vi "Batch Load Data.vi"(8 "Y Array Input":dbl[][](array[numeric])=array1024x10[10240 elements] format="%.2f") -> (2 "Data Array output":dbl[][](array[numeric])=[[156320.0], [157260.0], [158740.0], [160150.0], [162530.0], [164140.0], [166060.0], [167590.0], [169200.0], [171260.0], [172690.0], [174810.0], [176260.0], [178620.0], [180480.0], [181740.0], [183460.0], [185700.0], [187270.0], [189260.0], [191040.0], [192940.0], [193980.0], [196750.0], [198840.0], [200170.0], [202190.0], [203860.0], [205040.0], [206430.0], [209340.0], [210440.0], [213240.0], [214740.0], [216720.0], [218710.0], [220610.0], [222540.0], [224090.0], [226040.0], [227760.0], [228770.0], [231810.0], [233660.0], [235500.0], [237390.0], [239590.0], [241700.0], [243190.0], [245260.0], [245670.0], [248540.0], [250180.0], [252160.0], [254040.0], [255810.0], [257360.0], [258980.0], [260540.0], [261970.0], [262240.0], [265810.0], [266800.0], [268760.0], [270660.0], [271180.0], [273130.0], [274420.0], [276410.0], [276090.0], [278520.0], [280230.0], [281030.0], [281870.0], [283440.0], [285750.0], [286320.0], [287530.0], [288750.0], [288670.0], [290950.0], [292320.0], [293710.0], [294870.0], [295370.0], [296240.0], [297700.0], [298710.0], [298800.0], [301150.0], [302130.0], [303180.0], [303690.0], [304680.0], [305540.0], [306660.0], [307720.0], [308220.0], [307800.0], [310510.0], [310980.0], [311540.0], [312460.0], [312990.0], [313790.0], [314260.0], [315080.0], [314160.0], [316990.0], [317280.0], [317390.0], [317810.0], [318990.0], [319270.0], [319920.0], [320880.0], [320580.0], [321670.0], [323440.0], [324260.0], [324090.0], [325340.0], [326440.0], [327880.0], [328190.0], [329450.0], [328800.0], [331840.0], [332880.0], [333390.0], [334690.0], [335400.0], [336540.0], [337530.0], [338800.0], [338680.0], [340000.0], [341080.0], [341600.0], [342840.0], [343390.0], [344390.0], [345420.0], [346090.0], [346340.0], [346460.0], [349550.0], [349420.0], [350670.0], [351070.0], [351930.0], [353120.0], [353520.0], [354520.0], [354640.0], [355380.0], [356380.0], [357290.0], [358190.0], [358930.0], [359670.0], [359540.0], [360830.0], [361900.0], [360600.0], [362480.0], [363660.0], [364070.0], [364740.0], [364990.0], [366060.0], [366930.0], [367780.0], [367940.0], [368640.0], [369950.0], [370430.0], [371320.0], [371730.0], [372740.0], [373400.0], [373890.0], [374850.0], [374640.0], [376240.0], [378000.0], [377860.0], [379380.0], [380050.0], [380630.0], [381640.0], [382180.0], [382230.0], [383250.0], [385270.0], [385380.0], [387220.0], [387590.0], [387980.0], [389810.0], [390380.0], [391030.0], [390020.0], [392370.0], [393610.0], [394220.0], [394720.0], [395770.0], [397090.0], [397800.0], [398480.0], [398130.0], [399860.0], [400870.0], [401860.0], [402070.0], [403020.0], [404320.0], [405070.0], [406210.0], [407160.0], [406140.0], [408920.0], [410760.0], [410970.0], [412260.0], [413420.0], [414890.0], [415800.0], [416960.0], [417480.0], [417970.0], [420910.0], [421760.0], [422450.0], [425020.0], [425520.0], [427330.0], [429060.0], [430200.0], [429790.0], [433380.0], [434550.0], [435800.0], [437460.0], [439590.0], [441200.0], [442140.0], [444010.0], [444080.0], [447490.0], [449670.0], [449930.0], [451710.0], [453330.0], [454340.0], [456010.0], [459020.0], [459170.0], [459650.0], [463490.0], [464920.0], [466220.0], [467140.0], [469790.0], [470470.0], [471550.0], [473460.0], [473170.0], [476510.0], [478130.0], [479950.0], [481700.0], [482610.0], [484720.0], [486310.0], [487360.0], [488710.0], [488480.0], [491530.0], [493680.0], [494030.0], [496330.0], [496710.0], [499040.0], [500660.0], [502060.0], [501750.0], [505120.0], [507080.0], [509080.0], [510410.0], [511400.0], [513950.0], [515830.0], [516880.0], [518020.0], [517880.0], [521810.0], [522630.0], [524040.0], [526020.0], [526400.0], [527650.0], [529510.0], [531110.0], [530100.0], [534120.0], [534870.0], [536820.0], [537820.0], [538610.0], [539780.0], [542010.0], [541950.0], [543990.0], [542980.0], [545900.0], [546330.0], [547660.0], [548080.0], [549810.0], [550340.0], [551570.0], [553330.0], [551440.0], [554700.0], [555680.0], [557650.0], [558440.0], [559220.0], [559960.0], [561330.0], [562400.0], [562300.0], [561740.0], [564550.0], [565120.0], [566410.0], [566540.0], [567600.0], [569260.0], [569370.0], [570620.0], [569700.0], [573110.0], [574280.0], [574450.0], [575220.0], [576960.0], [577570.0], [580100.0], [580380.0], [581520.0], [581380.0], [585270.0], [586540.0], [587260.0], [589060.0], [590240.0], [591500.0], [593040.0], [594340.0], [593420.0], [596370.0], [597700.0], [598570.0], [601150.0], [601800.0], [604910.0], [606790.0], [607480.0], [608140.0], [609520.0], [612450.0], [613670.0], [614660.0], [615130.0], [616330.0], [617050.0], [618050.0], [620390.0], [620190.0], [624180.0], [625540.0], [626790.0], [628820.0], [629000.0], [630620.0], [631500.0], [632660.0], [632820.0], [635130.0], [637650.0], [638560.0], [639160.0], [640430.0], [641030.0], [642840.0], [644020.0], [644840.0], [643680.0], [646820.0], [648710.0], [649660.0], [649440.0], [650920.0], [652720.0], [653450.0], [654620.0], [654780.0], [656430.0], [657460.0], [657570.0], [659320.0], [659400.0], [660680.0], [661770.0], [662130.0], [662360.0], [661080.0], [664420.0], [664320.0], [665300.0], [665760.0], [665580.0], [666220.0], [667220.0], [667340.0], [666260.0], [666190.0], [667200.0], [666770.0], [667620.0], [667530.0], [667110.0], [667250.0], [666860.0], [666590.0], [664350.0], [667200.0], [666880.0], [666520.0], [666110.0], [665080.0], [664700.0], [665990.0], [664640.0], [663420.0], [662240.0], [662810.0], [663050.0], [662600.0], [662030.0], [662160.0], [660780.0], [660130.0], [657870.0], [655800.0], [658220.0], [657800.0], [655630.0], [654120.0], [654570.0], [652660.0], [652060.0], [651740.0], [649510.0], [647850.0], [647320.0], [646010.0], [644610.0], [642420.0], [640220.0], [640340.0], [638990.0], [637100.0], [633820.0], [634320.0], [632920.0], [631980.0], [630800.0], [629090.0], [628850.0], [627160.0], [625590.0], [623130.0], [621440.0], [621550.0], [620700.0], [618500.0], [617880.0], [616220.0], [615470.0], [612630.0], [611170.0], [607430.0], [608600.0], [606890.0], [604420.0], [603270.0], [601590.0], [599460.0], [597450.0], [596090.0], [592650.0], [591760.0], [591090.0], [589220.0], [586320.0], [586060.0], [584040.0], [581410.0], [580850.0], [578450.0], [574310.0], [574760.0], [572940.0], [570980.0], [569590.0], [567810.0], [565600.0], [563760.0], [561900.0], [557600.0], [557220.0], [554640.0], [552400.0], [551480.0], [549700.0], [548050.0], [546890.0], [545140.0], [542510.0], [538000.0], [538080.0], [536770.0], [534010.0], [531830.0], [530640.0], [529320.0], [527240.0], [525000.0], [520960.0], [521070.0], [520170.0], [518210.0], [516210.0], [515020.0], [512950.0], [511720.0], [510620.0], [508390.0], [503950.0], [504510.0], [503570.0], [501270.0], [500230.0], [498290.0], [497320.0], [496810.0], [493930.0], [490820.0], [491560.0], [489960.0], [489310.0], [486820.0], [485200.0], [484360.0], [481680.0], [480350.0], [478600.0], [474800.0], [474770.0], [472460.0], [471520.0], [469300.0], [467320.0], [465240.0], [463430.0], [461630.0], [456970.0], [457570.0], [455660.0], [453120.0], [450930.0], [448980.0], [446190.0], [444850.0], [443350.0], [441040.0], [436880.0], [436140.0], [434420.0], [432330.0], [430310.0], [428480.0], [426040.0], [424900.0], [422610.0], [419380.0], [418430.0], [416630.0], [416290.0], [414300.0], [412500.0], [411400.0], [410060.0], [408660.0], [407070.0], [403290.0], [403090.0], [401900.0], [400240.0], [399050.0], [397450.0], [395580.0], [394440.0], [393710.0], [390260.0], [390640.0], [388280.0], [386530.0], [385640.0], [384440.0], [382570.0], [381800.0], [381000.0], [378720.0], [377390.0], [376850.0], [375200.0], [374320.0], [373100.0], [371220.0], [370010.0], [368870.0], [367560.0], [364680.0], [364510.0], [363130.0], [361300.0], [360060.0], [358740.0], [357360.0], [355990.0], [354730.0], [352870.0], [351670.0], [351570.0], [350560.0], [349430.0], [349280.0], [348110.0], [348810.0], [348240.0], [347840.0], [346100.0], [347600.0], [347650.0], [348340.0], [348530.0], [348790.0], [348900.0], [348490.0], [349230.0], [348620.0], [347720.0], [349040.0], [348820.0], [348160.0], [348370.0], [348810.0], [348410.0], [348440.0], [348090.0], [346440.0], [347530.0], [347510.0], [347190.0], [346980.0], [346970.0], [347380.0], [346650.0], [346660.0], [346160.0], [345540.0], [346110.0], [346250.0], [346100.0], [346130.0], [345360.0], [345870.0], [346100.0], [345550.0], [344440.0], [345530.0], [345280.0], [345730.0], [345620.0], [345010.0], [345010.0], [345170.0], [345320.0], [343740.0], [344220.0], [345060.0], [344330.0], [345130.0], [344780.0], [344760.0], [344580.0], [344900.0], [344560.0], [343020.0], [343620.0], [343590.0], [343780.0], [342910.0], [343500.0], [343130.0], [343920.0], [343120.0], [342650.0], [342610.0], [343040.0], [343040.0], [342780.0], [342740.0], [342160.0], [341750.0], [341210.0], [340920.0], [339020.0], [340380.0], [339050.0], [338350.0], [337570.0], [337100.0], [336350.0], [335800.0], [335510.0], [333940.0], [333380.0], [334120.0], [334050.0], [333630.0], [334510.0], [334900.0], [335700.0], [337260.0], [338810.0], [339090.0], [343020.0], [345650.0], [347530.0], [350990.0], [354050.0], [357380.0], [360650.0], [363900.0], [365580.0], [369540.0], [373470.0], [375250.0], [377750.0], [379810.0], [381750.0], [383410.0], [384500.0], [386600.0], [385600.0], [387930.0], [389910.0], [390520.0], [391700.0], [392050.0], [391960.0], [391730.0], [392450.0], [390690.0], [393050.0], [392850.0], [393580.0], [394080.0], [392820.0], [393180.0], [392870.0], [392970.0], [393260.0], [390860.0], [391510.0], [391330.0], [390430.0], [389300.0], [388920.0], [388670.0], [388150.0], [388100.0], [386960.0], [388040.0], [388650.0], [387730.0], [387970.0], [386880.0], [387000.0], [386420.0], [386990.0], [385910.0], [383510.0], [384780.0], [384030.0], [384080.0], [383180.0], [381830.0], [381580.0], [381410.0], [381920.0], [379820.0], [381400.0], [381260.0], [381480.0], [381220.0], [381160.0], [380220.0], [379490.0], [379530.0], [379140.0], [377530.0], [378270.0], [377830.0], [377610.0], [376940.0], [376510.0], [376080.0], [375890.0], [376230.0], [373670.0], [374800.0], [374290.0], [373960.0], [373110.0], [373330.0], [372760.0], [371680.0], [371860.0], [371300.0], [367850.0], [368940.0], [368290.0], [367740.0], [367630.0], [366490.0], [366590.0], [365400.0], [364700.0], [362360.0], [362780.0], [362460.0], [361600.0], [361410.0], [360710.0], [359930.0], [359220.0], [358090.0], [358030.0], [355680.0], [356970.0], [355700.0], [355970.0], [355130.0], [354980.0], [354470.0], [354120.0], [353610.0], [351920.0], [353430.0], [353730.0], [353240.0], [352810.0], [352730.0], [352930.0], [353230.0], [352990.0], [352320.0], [352370.0], [353100.0], [353530.0], [354110.0], [353310.0], [354720.0], [354820.0], [355090.0], [356000.0], [354730.0], [356760.0], [357560.0], [358070.0], [358370.0], [359300.0], [359980.0], [361140.0], [362240.0], [362300.0], [362850.0], [364220.0], [365530.0], [366740.0], [367400.0], [368790.0], [369320.0], [370690.0], [372240.0], [370660.0], [374080.0], [374970.0], [376000.0], [377270.0], [378520.0], [379880.0], [381660.0], [383190.0], [384070.0], [384140.0], [386260.0], [388280.0], [389600.0], [391170.0], [392920.0], [393800.0], [395680.0], [397070.0], [397120.0], [400470.0], [401730.0], [403790.0], [406060.0], [406910.0], [408630.0], [411080.0], [413560.0], [413080.0], [415620.0], [418270.0], [419420.0], [421620.0], [423980.0], [426180.0], [427900.0], [429930.0], [431090.0], [432040.0], [435340.0], [437000.0], [439230.0], [441180.0], [442820.0], [445160.0], [447410.0], [448810.0], [450420.0], [452100.0], [453960.0], [456590.0], [457360.0], [460200.0], [462210.0], [464290.0], [466050.0], [467300.0], [467040.0], [470870.0], [472490.0], [475020.0], [476600.0], [479850.0], [481770.0], [483830.0], [485770.0], [487240.0], [489490.0], [491690.0], [493030.0], [495820.0], [497760.0], [499750.0], [502150.0], [504600.0], [507830.0], [505690.0], [510100.0], [512330.0], [514740.0], [516420.0], [517990.0], [520020.0], [521630.0], [523580.0], [524160.0], [525290.0], [528610.0], [529240.0], [531820.0], [533720.0], [536570.0], [537640.0], [539530.0], [541010.0], [542030.0], [545080.0], [547040.0], [548830.0], [550910.0], [551940.0], [553730.0], [556100.0], [556780.0], [557540.0], [560360.0], [562490.0], [563420.0], [565890.0], [565840.0], [556840.0]] format="%.2f")   [LabVIEW 2024]
doc: "This is a sub VI to load data into PlotBuffer.\nIt uses the x-arrayPlotBuffer (nm), data-arrayPlotBuffer and FileInfoBuffer as input and output. \nIt should be used in a shift-register settings"
uses:
  Globals and TypeDefs/Type Definitions.llb/3 way Status.ctl
panel:
  in  "Cancel":bool
  in  "stop":bool
  in  "Select Files":i32[](listbox)
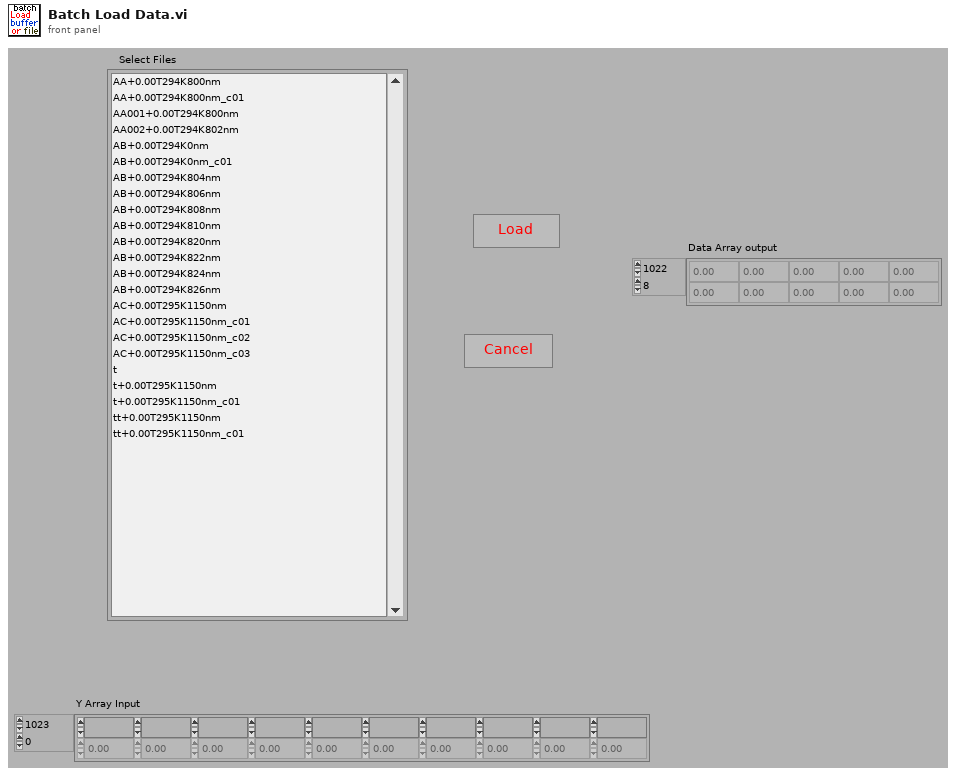
[diagram p1: front panel]
types:
  T1 = typedef "3 way Status.ctl" = u8
  T2 = enum32{"existing file", "new file", "new or existing file", "existing dir", "new dir", "new or existing dir", "existing file (use LLBs)", "new file (use LLBs)", "new or existing file (use LLBs)", "new or existing file or directory (use LLBs)"}
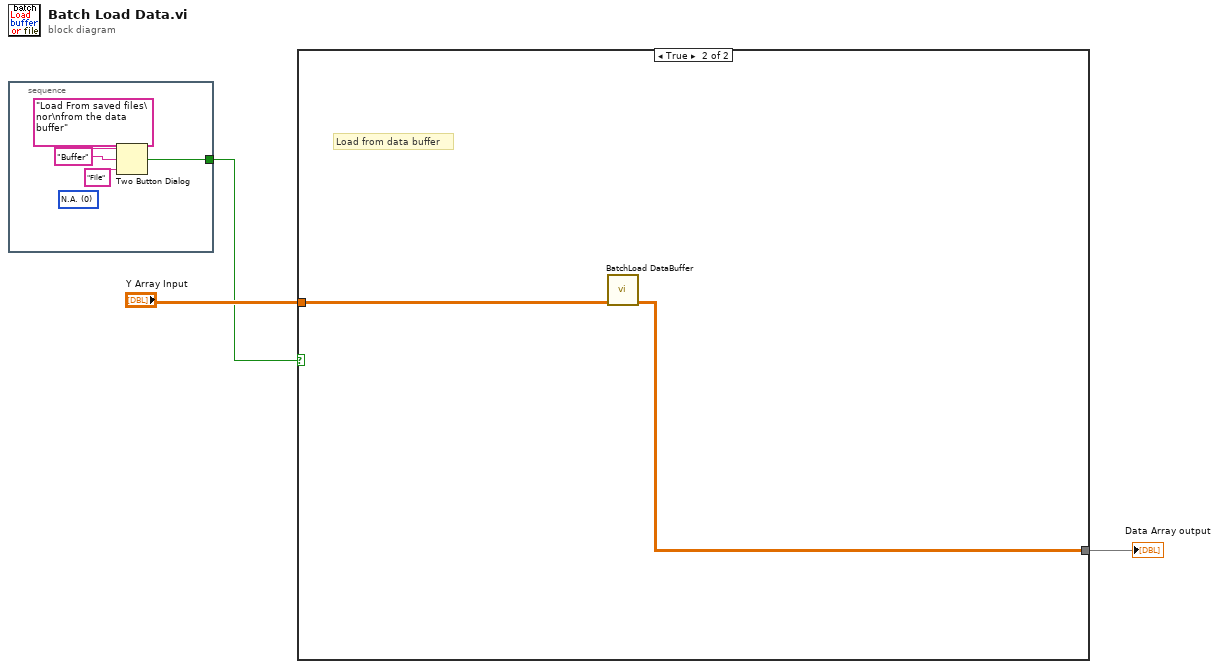
[diagram p0: block diagram]
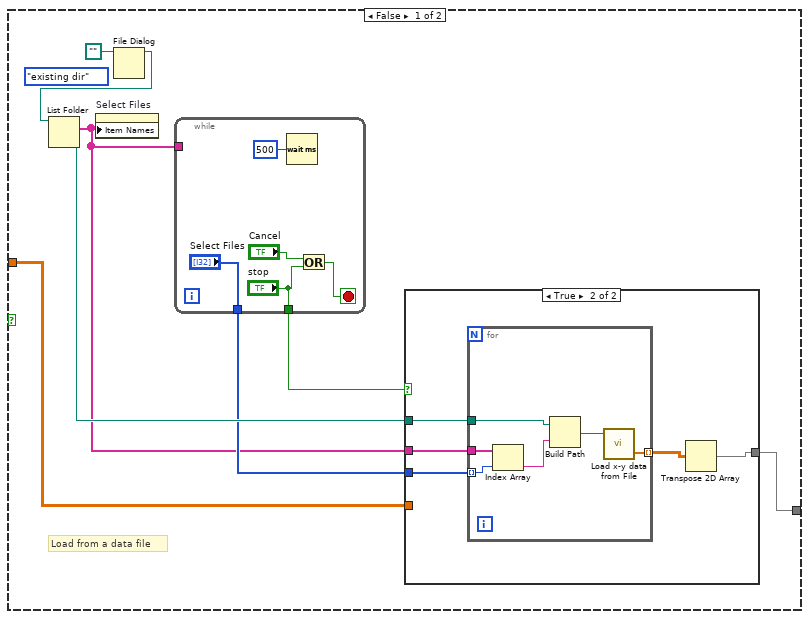
[diagram p2: hidden frame]
diagram:
  n1 = stacked-sequence {
    tunnel: [w7] -> w1
    frame #0 {
      (unwired) T1 0 items=["N.A.", "OK", "Busy", "Done"] ("Buffer")
      n2 = Two Button Dialog(message="Load From saved files\nor\nfrom the data buffer", 1:"File" ("F button name (\"Cancel\")"), 2:"Buffer" ("T button name (\"OK\")")) -> (T button?=w7:bool)
    }
  }
  n3 = case shown="True" w1 {
    tunnel: "Y Array Input" -> [w10 w33]
    tunnel: [w11 w34] -> w2
    frame False {
      (unwired) T2."existing dir" ("select mode (2)")
      # "Load from a data file"
      n4 = File Dialog(11:path "") -> (3:w8:path)  [unwired: 6 in, 3 out]
      n5 = List Folder(path=w8) -> (path out=w14:path, filenames=w12:string[])  [unwired: 3 in, 2 out]
      n6 = property on="Select Files" class="LstBox (strict)"("Item Names"=w12) -> ()  [unwired: 2 in, 2 out]
      n7 = while {
        tunnel: w12 -> [_]
        tunnel: ["stop"] -> w15
        tunnel: ["Select Files"] -> w13
        stop <- w31 stop-if-true
        n8 = Wait (ms)(milliseconds to wait=u32 500) -> ()  [unwired: 1 out]
        n9 = Or(x="Cancel", y="stop") -> (x .or. y?=w31:bool)
      }
      n10 = case shown="True" w15 {
        tunnel: w14 -> [_ w19]
        tunnel: w13 -> [_ w21]
        tunnel: w12 -> [_ w20]
        tunnel: [w16 w17] -> w11
        tunnel: w10 -> [w16 _]
        frame False {
        }
        frame True {
          n11 = for {
            tunnel: w21 -> [w26] mode=indexing
            tunnel: w20 -> [w27]
            tunnel: w19 -> [w25]
            tunnel: [w22] -> w18 mode=indexing
            n12 = Index Array(array=w27, index=w26) -> (element=w24:string)
            n13 = Build Path(base path=w25, name or relative path=w24) -> (appended path=w23:path)
            n14 = call "Load x-y data from File.vi"("file path"=w23) -> ("Y-Array"=w22:sgl[])  [unwired: 2 in, 1 out]
          }
          n15 = Transpose 2D Array(2D array=w18) -> (transposed array=w17:sgl[][])
        }
      }
    }
    frame True {
      # "Load from data buffer"
      n16 = call "BatchLoad DataBuffer.vi"("Y Array In"=w33) -> ("Y Array Out"=w34:dbl[][])  [unwired: 8 in, 6 out]
    }
  }
  "Data Array output" <- w2
